vi "VideoStreamTest.vi"() -> ()   [LabVIEW 2022 SP3]
uses:
  <vilib>/userdefined/High Color/IMAQdx.ctl
  <vilib>/vision/driver/NI_Vision_Acquisition_Software.lvlib
panel:
  out "Image":T1(plugin-control)
  in  "stop":bool
  in  "Session In 3":T2
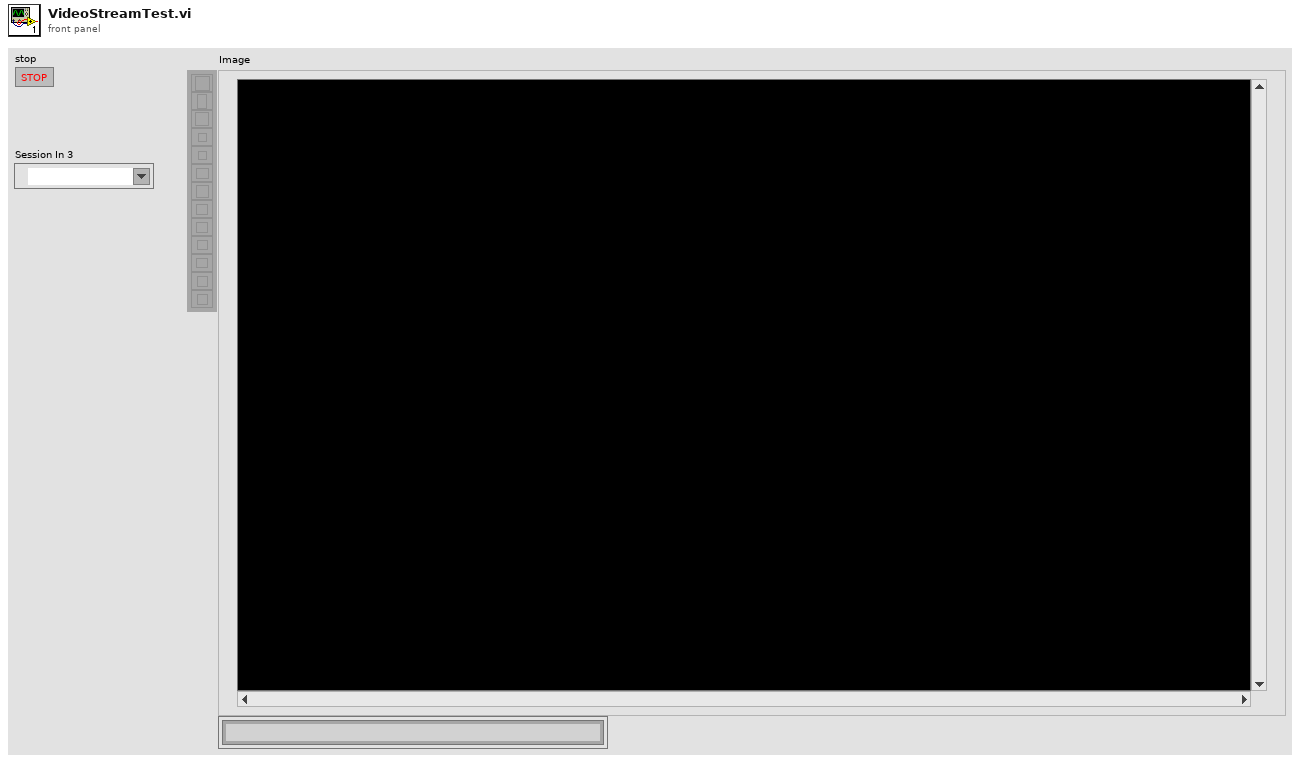
[diagram p1: front panel]
types:
  T1 = typedef "IMAQ Image.ctl" = refnum<image>
  T2 = typedef "IMAQdx.ctl" = refnum<k21>
  T3 = typedef "Image Type" = u32
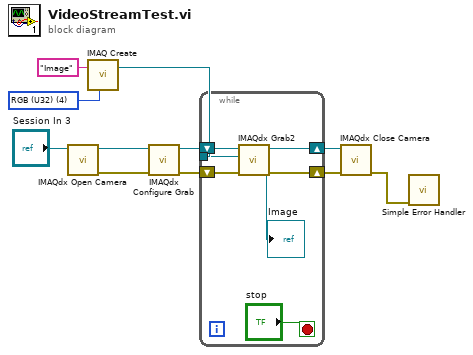
[diagram p0: block diagram]
diagram:
  w3 = T3 4 items=["Grayscale (U8)", "Grayscale (I16)", "Grayscale (SGL)", "Complex (CSG)", "RGB (U32)", "HSL (U32)", "RGB (U64)", "Grayscale (U16)"] ("Image Type")
  n1 = call <vilib>:"IMAQdx Open Camera.vi"("Session In"="Session In 3") -> ("error out"=w7:errorcluster, "Session Out"=w10:T2)  [unwired: 9 in]
  n2 = call "IMAQ Create"("Image Name"="Image", "Image Type"=w3) -> ("New Image"=w2:T1)  [unwired: 3 in, 1 out]
  n3 = call <vilib>:"IMAQdx Configure Grab.vi"("error in"=w7, "Session In"=w10) -> ("error out"=w6:errorcluster, "Session Out"=w9:T2)  [unwired: 8 in]
  n4 = while {
    tunnel: w2 -> [w14]
    shift-right: [w17] -> w8
    shift-left: w9 -> [w18]
    shift-right: [w15] -> w5
    shift-left: w6 -> [w16]
    stop <- "stop" stop-if-true
    n5 = call <vilib>:"IMAQdx Grab2.vi"("error in"=w16, "Image In"=w14, "Session In"=w18) -> ("error out"=w15:errorcluster, "Image Out"=→"Image":T1, "Session Out"=w17:T2)  [unwired: 5 in, 1 out]
  }
  n6 = call <vilib>:"IMAQdx Close Camera.vi"("error in"=w5, "Session In"=w8) -> ("error out"=w1:errorcluster)  [unwired: 9 in]
  n7 = call <vilib>:"Simple Error Handler.vi"("error in (no error)"=w1) -> ()  [unwired: 4 in, 5 out]
